vi "_Axis Value.vi"(8 "error in (no error)":errorcluster, 10 "Index":i32, 11 "Joystick in":refnum<class "Joystick.lvclass">) -> (0 "error out":errorcluster, 2 "Value":dbl, 3 "Joystick out":refnum<class "Joystick.lvclass">)   [LabVIEW 2020, in "Joystick.lvlib" / "Joystick.lvclass"]
uses:
  Joystick.lvclass
  Joystick.lvclass/Joystick.ctl
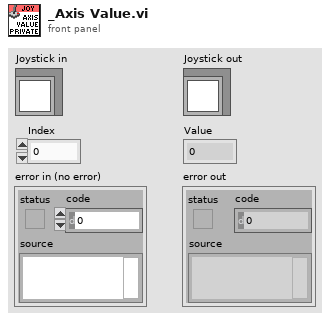
[diagram p1: front panel]
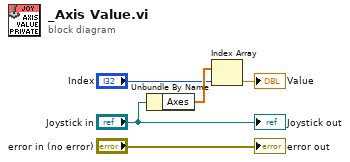
[diagram p0: block diagram]
diagram:
  n1 = Unbundle By Name("Joystick in") -> ("Axes"=w4:dbl[])
  n2 = Index Array(array=w4, index="Index") -> (element=→"Value":dbl)
  "error out" <- "error in (no error)"
  "Joystick out" <- "Joystick in"
